vi "GPS.vi"() -> ()   [LabVIEW 2020]
panel:
  out "mod indicador + cheksum":string
  out "direccion magnetica":string
  out "variacion magnetica":string
  out "fecha":string
  out "direccion del viento":string
  out "velocidad del viento":string
  out "direccion longitud":string
  out "longitud":string
  out "direccion latitud":string
  out "latitud":string
  out "status":string
  out "hora":string
  out "identificador de tipo de trama":string
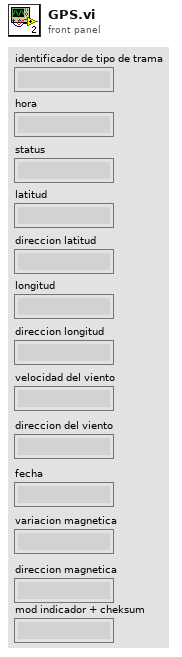
[diagram p1: front panel]
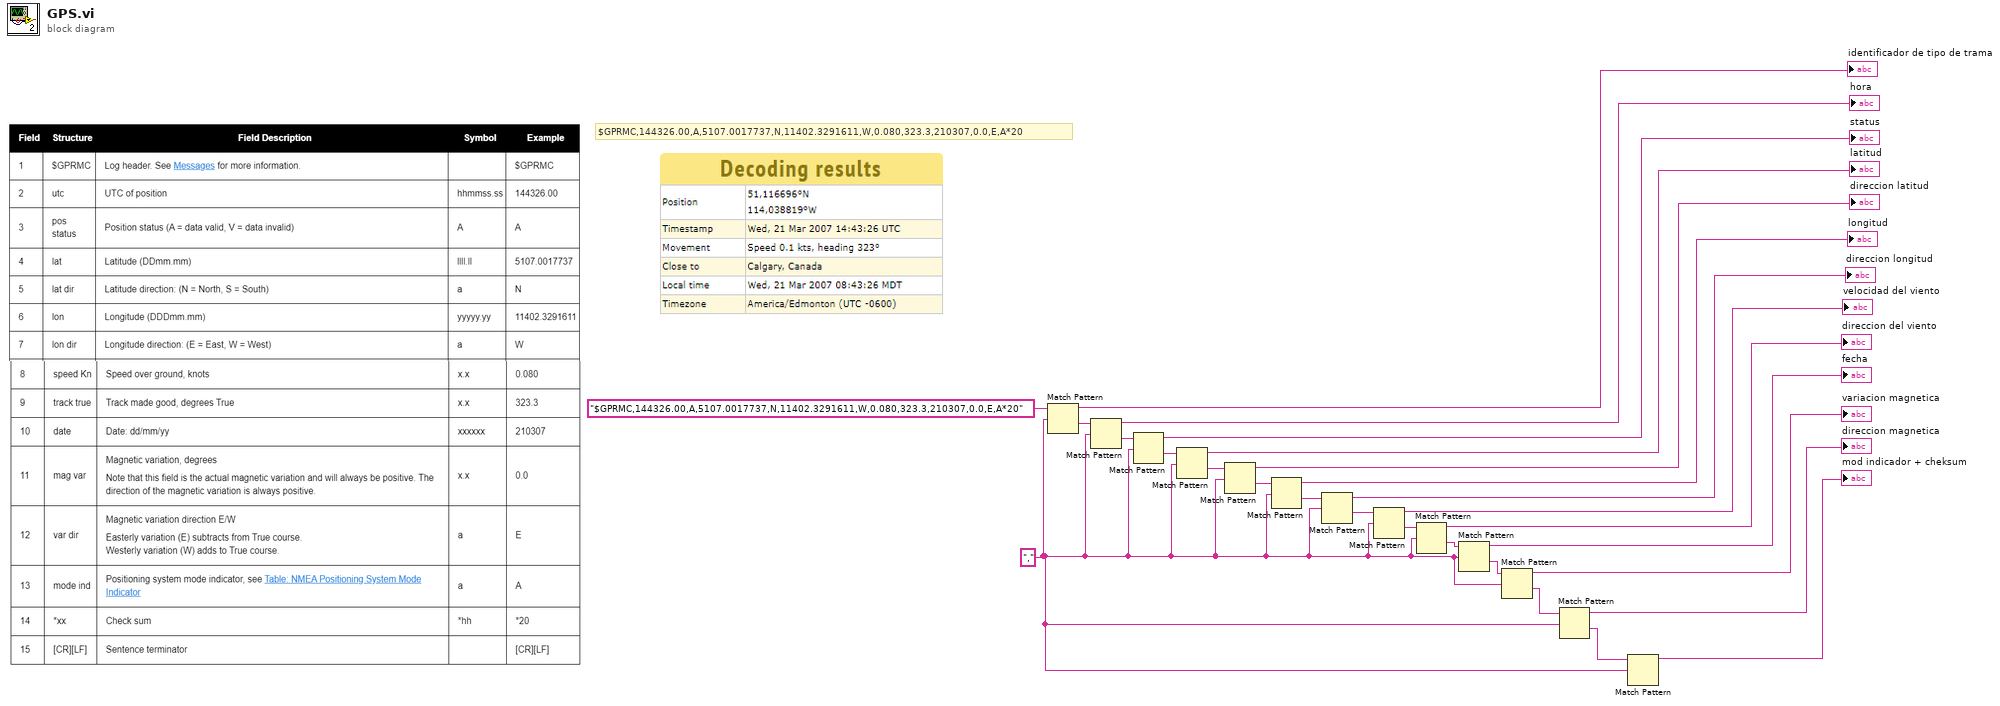
[diagram p0: block diagram]
diagram:
  w2 = "," ("regular expression")
  # "$GPRMC,144326.00,A,5107.0017737,N,11402.3291611,W,0.080,323.3,210307,0.0,E,A*20"
  n1 = Match Pattern(string="$GPRMC,144326.00,A,5107.0017737,N,11402.3291611,W,0.080,323.3,210307,0.0,E,A*20", regular expression=w2) -> (before substring=→"identificador de tipo de trama":string, after substring=w25:string)  [unwired: 1 in, 2 out]
  n2 = Match Pattern(string=w25, regular expression=w2) -> (before substring=→"hora":string, after substring=w23:string)  [unwired: 1 in, 2 out]
  n3 = Match Pattern(string=w23, regular expression=w2) -> (before substring=→"status":string, after substring=w21:string)  [unwired: 1 in, 2 out]
  n4 = Match Pattern(string=w21, regular expression=w2) -> (before substring=→"latitud":string, after substring=w19:string)  [unwired: 1 in, 2 out]
  n5 = Match Pattern(string=w19, regular expression=w2) -> (before substring=→"direccion latitud":string, after substring=w17:string)  [unwired: 1 in, 2 out]
  n6 = Match Pattern(string=w17, regular expression=w2) -> (before substring=→"longitud":string, after substring=w15:string)  [unwired: 1 in, 2 out]
  n7 = Match Pattern(string=w15, regular expression=w2) -> (before substring=→"direccion longitud":string, after substring=w13:string)  [unwired: 1 in, 2 out]
  n8 = Match Pattern(string=w13, regular expression=w2) -> (before substring=→"velocidad del viento":string, after substring=w11:string)  [unwired: 1 in, 2 out]
  n9 = Match Pattern(string=w11, regular expression=w2) -> (before substring=→"direccion del viento":string, after substring=w9:string)  [unwired: 1 in, 2 out]
  n10 = Match Pattern(string=w9, regular expression=w2) -> (before substring=→"fecha":string, after substring=w7:string)  [unwired: 1 in, 2 out]
  n11 = Match Pattern(string=w7, regular expression=w2) -> (before substring=→"variacion magnetica":string, after substring=w5:string)  [unwired: 1 in, 2 out]
  n12 = Match Pattern(string=w5, regular expression=w2) -> (before substring=→"direccion magnetica":string, after substring=w3:string)  [unwired: 1 in, 2 out]
  n13 = Match Pattern(string=w3, regular expression=w2) -> (before substring=→"mod indicador + cheksum":string)  [unwired: 1 in, 3 out]
